vi "check fns availability.vi"(8 "error in (no error)":errorcluster, 10 "fns list is":string[](array[string])) -> (0 "error out":errorcluster, 1 "unavailable fns":string[](array[string]), 2 "available fns":string[](array[string]), 3 "all available":bool, 4 "Jl Server state out":T1, 5 "return code":u8, 6 "detailed error info":T2)   [LabVIEW 2018, in "LV-0mq-Julia_roundtrip-lib.lvlib"]
uses:
  LV-0mq-Julia_roundtrip-lib.lvlib
  detailed error info.ctl
  StackFrame.ctl
  Server or client state.ctl
  <vilib>/Utility/error.llb/Error Cluster From Error Code.vi
  <vilib>/ErrorRing/Error Ring.xnode
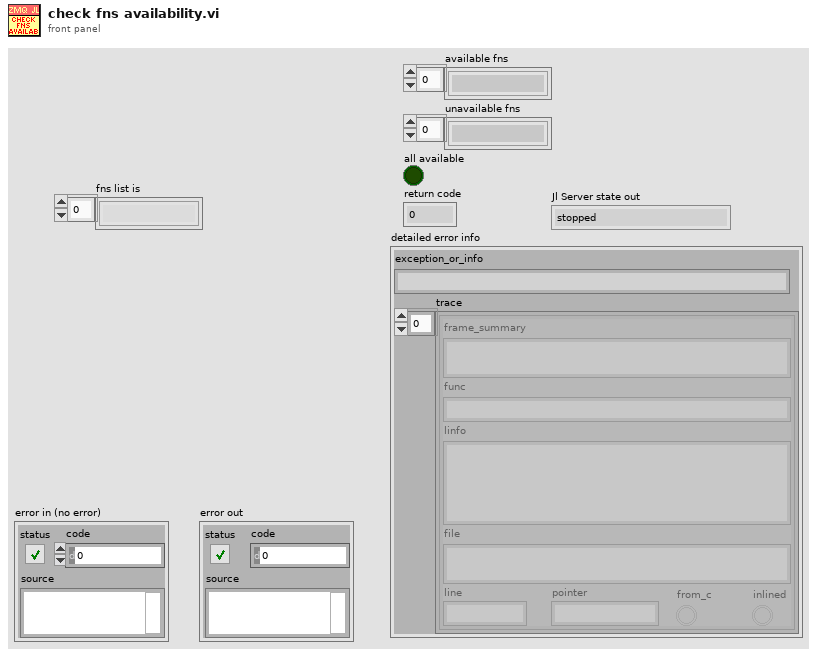
[diagram p1: front panel]
types:
  T1 = typedef "LV-0mq-Julia_roundtrip-lib.lvlib/Server or client state.ctl" = enum16{"stopped", "running", "unknown"}
  T2 = typedef "LV-0mq-Julia_roundtrip-lib.lvlib/detailed error info.ctl" = cluster{"exception_or_info":string, "trace":T3[]}
  T3 = typedef "LV-0mq-Julia_roundtrip-lib.lvlib/StackFrame.ctl" = cluster{"frame_summary":string, "func":string, "linfo":string, "file":string, "line":i32, "pointer":u64, "from_c":bool, "inlined":bool}
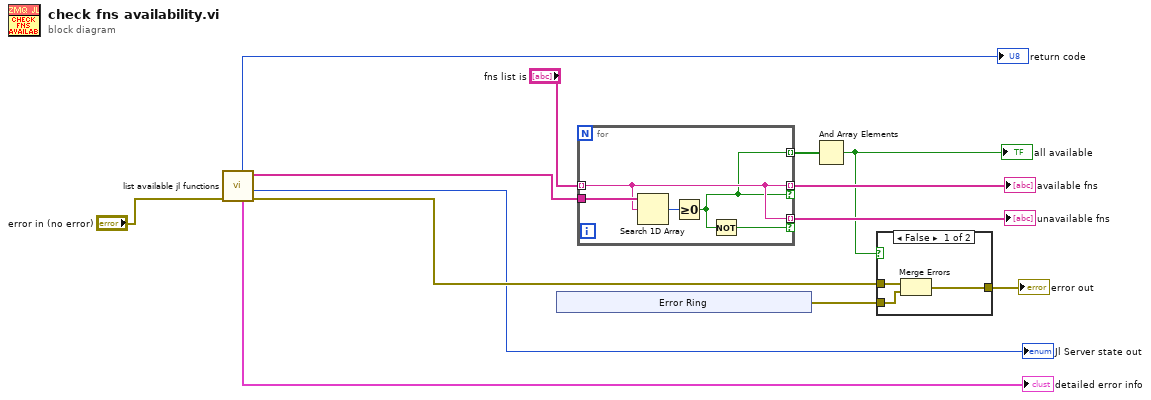
[diagram p0: block diagram]
diagram:
  n1 = call "list available jl functions.vi"("error in (no error)"="error in (no error)") -> ("error out"=w13:errorcluster, "Jl Server state out"=→"Jl Server state out":T1, "ext_fns"=w1:string[], "detailed error info"=→"detailed error info":T2, "return code"=→"return code":u8)  [unwired: 6 in]
  n2 = xnode "Error Ring"() -> ("error out"=w5:errorcluster)
  n3 = for {
    tunnel: "fns list is" -> [w16] mode=indexing
    tunnel: w1 -> [w18]
    tunnel: [w16] -> w10 mode=indexing if=w14
    tunnel: [w16] -> w9 mode=indexing if=w15
    tunnel: [w14] -> w8 mode=indexing
    n4 = Search 1D Array(1D array=w18, element=w16) -> (index of element=w17:i32)  [unwired: 1 in]
    n5 = Greater Or Equal To 0?(x=w17) -> (x >= 0?=w14:bool)
    n6 = Not(x=w14) -> (.not. x?=w15:bool)
  }
  "available fns" <- w10
  "unavailable fns" <- w9
  n7 = And Array Elements(Boolean array=w8) -> (logical AND=w6:bool)
  "all available" <- w6
  n8 = case shown="False" w6 {
    tunnel: w13 -> [w21 w22]
    tunnel: [w20 w22] -> w7
    tunnel: w5 -> [w19 _]
    frame False {
      n9 = Merge Errors(w21, w19) -> (w20:errorcluster)
    }
    frame True {
    }
  }
  "error out" <- w7
